vi "exit.vi"(8 "error in (no error)":errorcluster, 11 "CameraManager in":refnum<class "CameraManager.lvclass">) -> (0 "error out":errorcluster, 3 "CameraManager out":refnum<class "CameraManager.lvclass">)   [LabVIEW 2009, in "iManagement.lvlib" / "CameraManager.lvclass"]
doc: "Exits the camera application"
uses:
  CameraManager.lvclass
  CameraManager.lvclass/CameraManager.ctl
  Hal/Channels/Camera/CameraController.lvclass
  Hal/Channels/Camera/CameraEventsManager/CameraEventsManger.lvclass
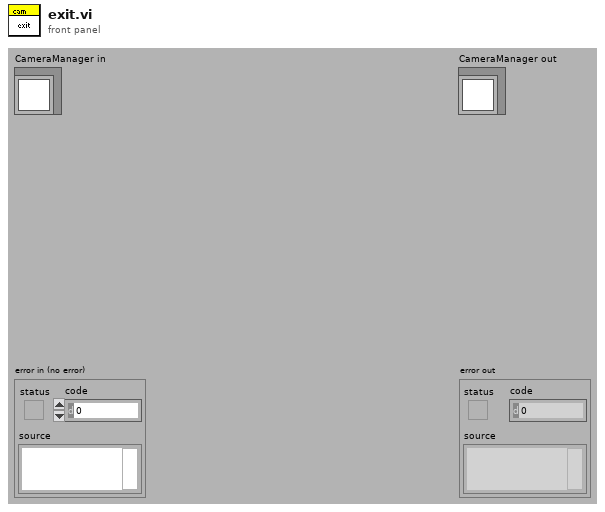
[diagram p1: front panel]
types:
  T1 = cluster{"closeEvent":refnum<user-event>, "temperatureUpdateEvent":refnum<user-event>, "displayErrorEvent":refnum<user-event>, "setPointUpdateEvent":refnum<user-event>}
  T2 = cluster{"newSetPointEvent":refnum<user-event>, "stopCoolingEvent":refnum<user-event>}
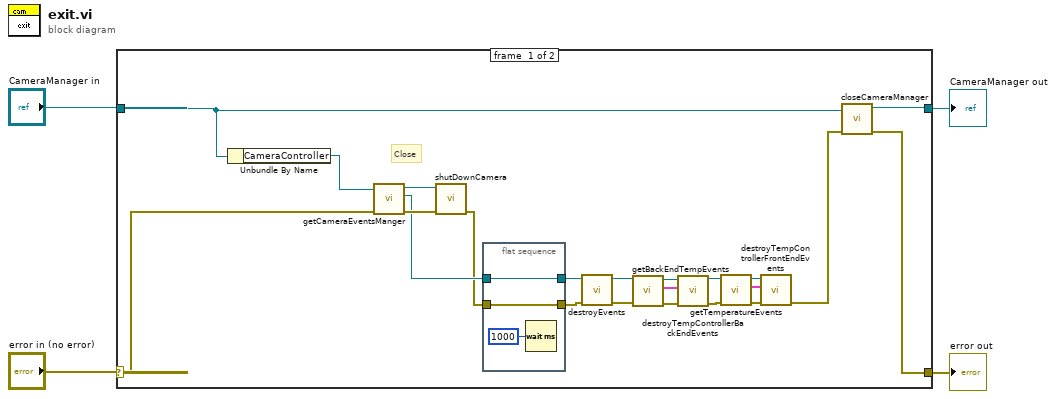
[diagram p0: block diagram]
diagram:
  n1 = case shown="No Error" "error in (no error)" {
    selector: "error in (no error)" -> [w9 w31]
    tunnel: [w14 w31] -> w3
    tunnel: [w16 w30] -> w1
    tunnel: "CameraManager in" -> [w10 w30]
    frame #0 {
      # "Close"
      n2 = Unbundle By Name(w10) -> ("CameraController"=w11:refnum<class "CameraController.lvclass">)
      n3 = call-dynamic "getCameraEventsManger.vi"("error in (no error)"=w9, "CameraController.lvclass in"=w11) -> ("error out"=w12:errorcluster, "Hardware:Channels.lvlib:CameraEventsManger.lvclass"=w7:refnum<class "CameraEventsManger.lvclass">, "CameraController.lvclass out"=w13:refnum<class "CameraController.lvclass">)  [unwired: 7 in]
      n4 = call-dynamic "shutDownCamera.vi"("error in (no error)"=w12, "CameraController in"=w13) -> ("error out"=w5:errorcluster)  [unwired: 7 in, 2 out]
      n5 = flat-sequence {
        tunnel: w7 -> [w29]
        tunnel: [w29] -> w8
        tunnel: [w28] -> w6
        tunnel: w5 -> [w28]
        frame #0 {
          n6 = Wait (ms)(milliseconds to wait=1000) -> ()  [unwired: 1 out]
        }
      }
      n7 = call-dynamic "destroyEvents.vi"("error in (no error)"=w6, "CameraEventsManger in"=w8) -> ("error out"=w25:errorcluster, "CameraEventsManger out"=w26:refnum<class "CameraEventsManger.lvclass">)  [unwired: 8 in]
      n8 = call-dynamic "getBackEndTempEvents.vi"("error in (no error)"=w25, "CameraEventsManger.lvclass in"=w26) -> ("error out"=w22:errorcluster, "backEndTempEvents"=w23:T1, "CameraEventsManger.lvclass out"=w24:refnum<class "CameraEventsManger.lvclass">)  [unwired: 7 in]
      n9 = call-dynamic "destroyTempControllerBackEndEvents.vi"("error in (no error)"=w22, "tempControllerBackEndEvents"=w23, "CameraEventsManger in"=w24) -> ("error out"=w20:errorcluster, "CameraEventsManger out"=w21:refnum<class "CameraEventsManger.lvclass">)  [unwired: 7 in]
      n10 = call-dynamic "getTemperatureEvents.vi"("error in (no error)"=w20, "CameraEventsManger.lvclass in"=w21) -> ("error out"=w19:errorcluster, "temperatureEvents"=w17:T2, "CameraEventsManger.lvclass out"=w18:refnum<class "CameraEventsManger.lvclass">)  [unwired: 7 in]
      n11 = call "destroyTempControllerFrontEndEvents.vi"("error in (no error)"=w19, "tempControllerFrontEndEvents"=w17, "CameraEventsManger in"=w18) -> ("error out"=w15:errorcluster)  [unwired: 7 in, 1 out]
      n12 = call "closeCameraManager.vi"("error in (no error)"=w15, "CameraManager in"=w10) -> ("error out"=w14:errorcluster, "CameraManager out"=w16:refnum<class "CameraManager.lvclass">)  [unwired: 8 in]
    }
    frame #1 {
    }
  }
  "error out" <- w3
  "CameraManager out" <- w1
